vi "Init GUI Objects.vi"(4 "Copy Error Details To Clipboard":refnum<vi>, 5 "Clipboard Confirmation Message":refnum<vi>, 6 "Module Init Timestamp":timestamp, 7 "Error Details":T1, 8 "Error In":errorcluster, 9 "Timestamp":refnum<vi>, 10 "Error Message":refnum<vi>, 11 "Error Code":refnum<vi>) -> (0 "Error Out":errorcluster)   [LabVIEW 2023, in "Error Manager.lvlib" / "Error Display Window.lvclass"]
doc: "This VI configures the \"look and feel\" of GUI objects, and sets their value (their contents)."
uses:
  Error Display Window.lvclass
  Error Details (cluster).ctl
  <vilib>/Utility/miscctls.llb/LVFontTypeDef.ctl
  Error Display Window.lvclass/Error Display Window.ctl
  Error Manager.lvlib
panel:
  # "Development\nControls or indicators that are useful for development or testing, but which are not outputs of the VI."
  # "Input\nInputs to the VI"
  # "Output\nOutputs of the VI"
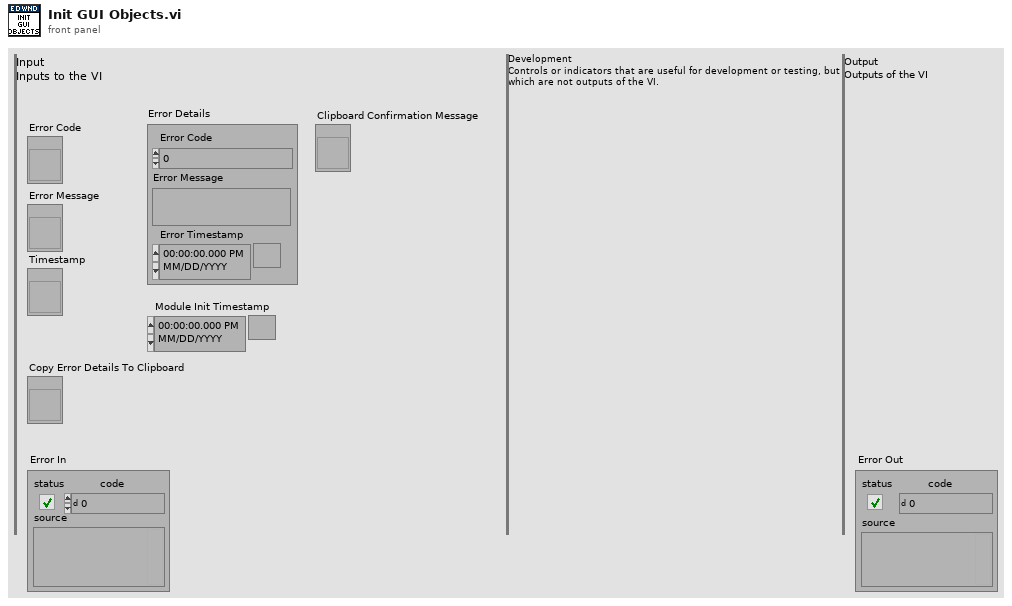
[diagram p1: front panel]
types:
  T1 = typedef "Error Manager.lvlib/Error Display Window.lvclass/Error Details (cluster).ctl" = cluster{"Error Code":i32, "Error Message":string, "Error Timestamp":timestamp}
  T2 = enum8{"Enabled", "Disabled", "Disabled and Grayed Out"}
  T3 = typedef "LVFontTypeDef.ctl" = cluster{"Font Name":string, "Size":u16, "Bold":bool, "Italic":bool, "Underline":bool, "Strikeout":bool, "Color":u32}
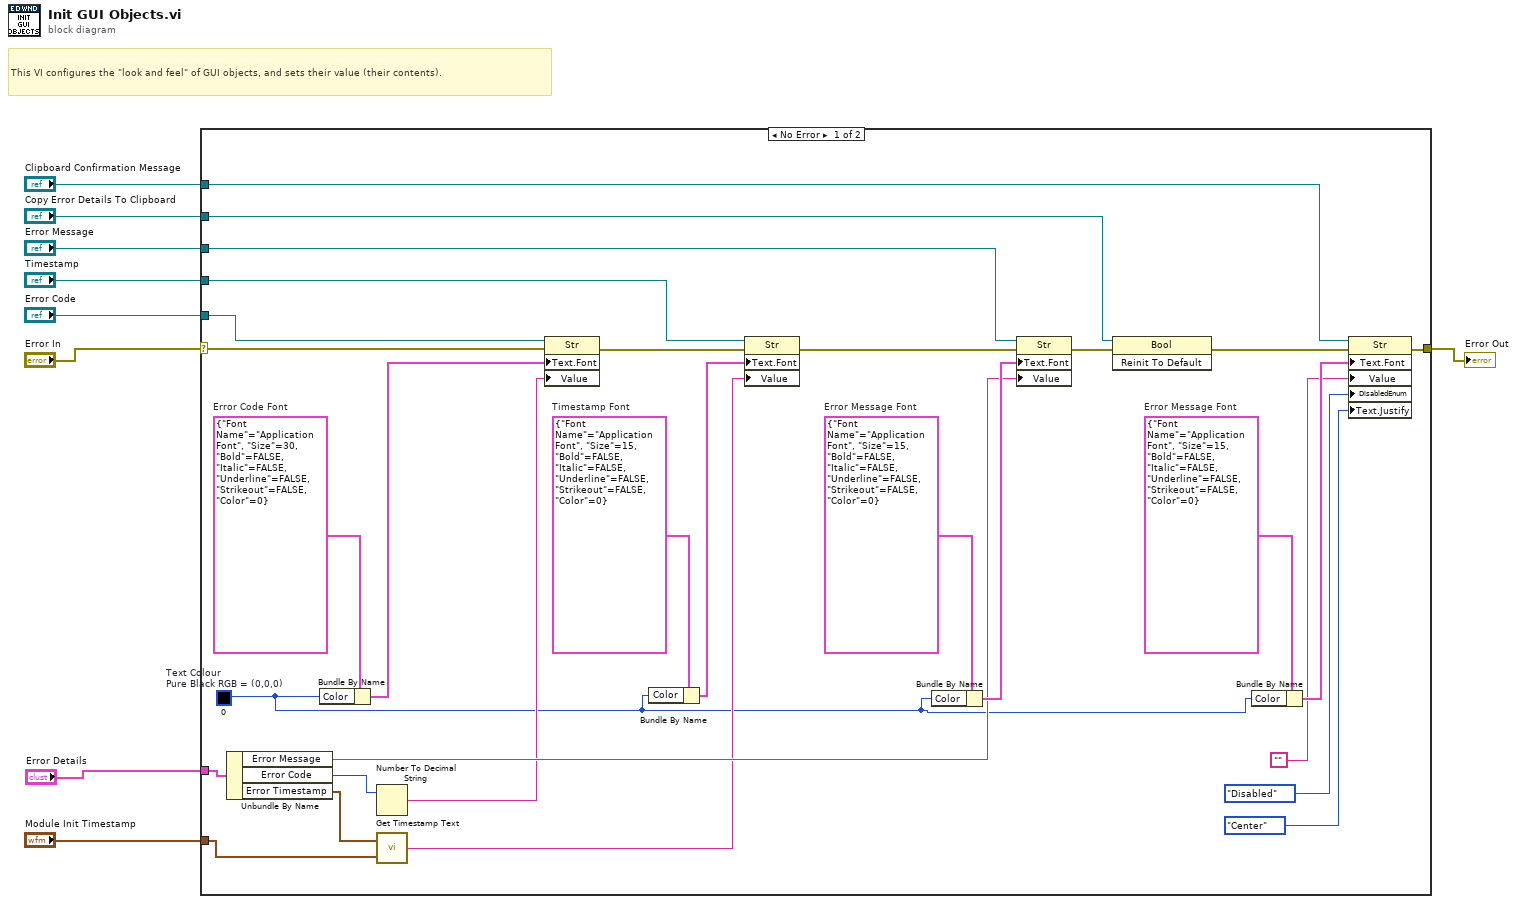
[diagram p0: block diagram]
diagram:
  # "This VI configures the \"look and feel\" of GUI objects, and sets their value (their contents)."
  n1 = case shown="No Error" "Error In" {
    selector: "Error In" -> [w39 w40]
    tunnel: [w15 w40] -> w8
    tunnel: "Error Code" -> [w38 _]
    tunnel: "Error Message" -> [w35 _]
    tunnel: "Error Details" -> [w36 _]
    tunnel: "Timestamp" -> [w25 _]
    tunnel: "Module Init Timestamp" -> [w21 _]
    tunnel: "Copy Error Details To Clipboard" -> [w19 _]
    tunnel: "Clipboard Confirmation Message" -> [w13 _]
    frame No Error {
      w17 = T3 {"Font Name"="Application Font", "Size"=15, "Bold"=FALSE, "Italic"=FALSE, "Underline"=FALSE, "Strikeout"=FALSE, "Color"=0}  # Error Message Font
      w24 = T3 {"Font Name"="Application Font", "Size"=15, "Bold"=FALSE, "Italic"=FALSE, "Underline"=FALSE, "Strikeout"=FALSE, "Color"=0}  # Timestamp Font
      w33 = T3 {"Font Name"="Application Font", "Size"=15, "Bold"=FALSE, "Italic"=FALSE, "Underline"=FALSE, "Strikeout"=FALSE, "Color"=0}  # Error Message Font
      w14 = u32 0  # Text Colour Pure Black RGB = (0,0,0)
      w37 = T3 {"Font Name"="Application Font", "Size"=30, "Bold"=FALSE, "Italic"=FALSE, "Underline"=FALSE, "Strikeout"=FALSE, "Color"=0}  # Error Code Font
      n2 = Unbundle By Name(w36) -> ("Error Message"=w31:string, "Error Code"=w29:i32, "Error Timestamp"=w22:timestamp)
      n3 = Bundle By Name(cluster=w37, "Color"=w14) -> (w30:T3)
      n4 = Number To Decimal String(number=w29) -> (decimal integer string=w28:string)  [unwired: 1 in]
      n5 = call "Get Timestamp Text.vi"("Module Init Timestamp"=w21, "Error Timestamp"=w22) -> ("Timestamp String"=w20:string)
      n6 = property class="Str"(reference=w38, error in=w39, "Text.Font"=w30, "Value"=w28) -> (error out=w27:errorcluster)  [unwired: 1 out]
      n7 = Bundle By Name(cluster=w24, "Color"=w14) -> (w23:T3)
      n8 = property class="Str"(reference=w25, error in=w27, "Text.Font"=w23, "Value"=w20) -> (error out=w26:errorcluster)  [unwired: 1 out]
      n9 = Bundle By Name(cluster=w33, "Color"=w14) -> (w32:T3)
      n10 = property class="Str"(reference=w35, error in=w26, "Text.Font"=w32, "Value"=w31) -> (error out=w34:errorcluster)  [unwired: 1 out]
      n11 = invoke class="Bool" method="Reinit To Default"(reference=w19, error in=w34) -> (error out=w16:errorcluster)  [unwired: 1 in, 2 out]
      n12 = Bundle By Name(cluster=w17, "Color"=w14) -> (w18:T3)
      n13 = property class="Str"(reference=w13, error in=w16, "Text.Font"=w18, "Value"="", "DisabledEnum"=T2."Disabled" ("Disabled"), "Text.Justify"=enum16{"Left", "Center", "Right"}."Center" ("Text.Justification")) -> (error out=w15:errorcluster)  [unwired: 1 out]
    }
    frame Error {
    }
  }
  "Error Out" <- w8
